vi "(SubVI)-Cut and Fit to Sutckbead-XY-QPD&BeadPosition_YCC.vi"(5 "Stuckbead path (dialog if empty)":path) -> (0 "Best Fit for Bead position (nm)":dbl[](array[numeric]), 1 "Cut-BeadPosition Array Out (nm)":dbl[](array[numeric]), 2 "Cut-QPD signal Out":dbl[](array[numeric]), 3 "All fig":T2(array[cluster]), 4 "Polynomial Coefficients\nx:QPD, y:BeadPos":dbl[](array[numeric]))   [LabVIEW 2014]
uses:
  <vilib>/Utility/file.llb/Read From Spreadsheet File (DBL).vi
  <vilib>/Analysis/NI_AALPro.lvlib
panel:
  out "XY Graph 2":T1(graph)
  out "XY Graph":T2(graph)
  out "stuckbead-QPD (V)":dbl[](array[numeric])
  out "Stage (um)":dbl[](array[numeric])
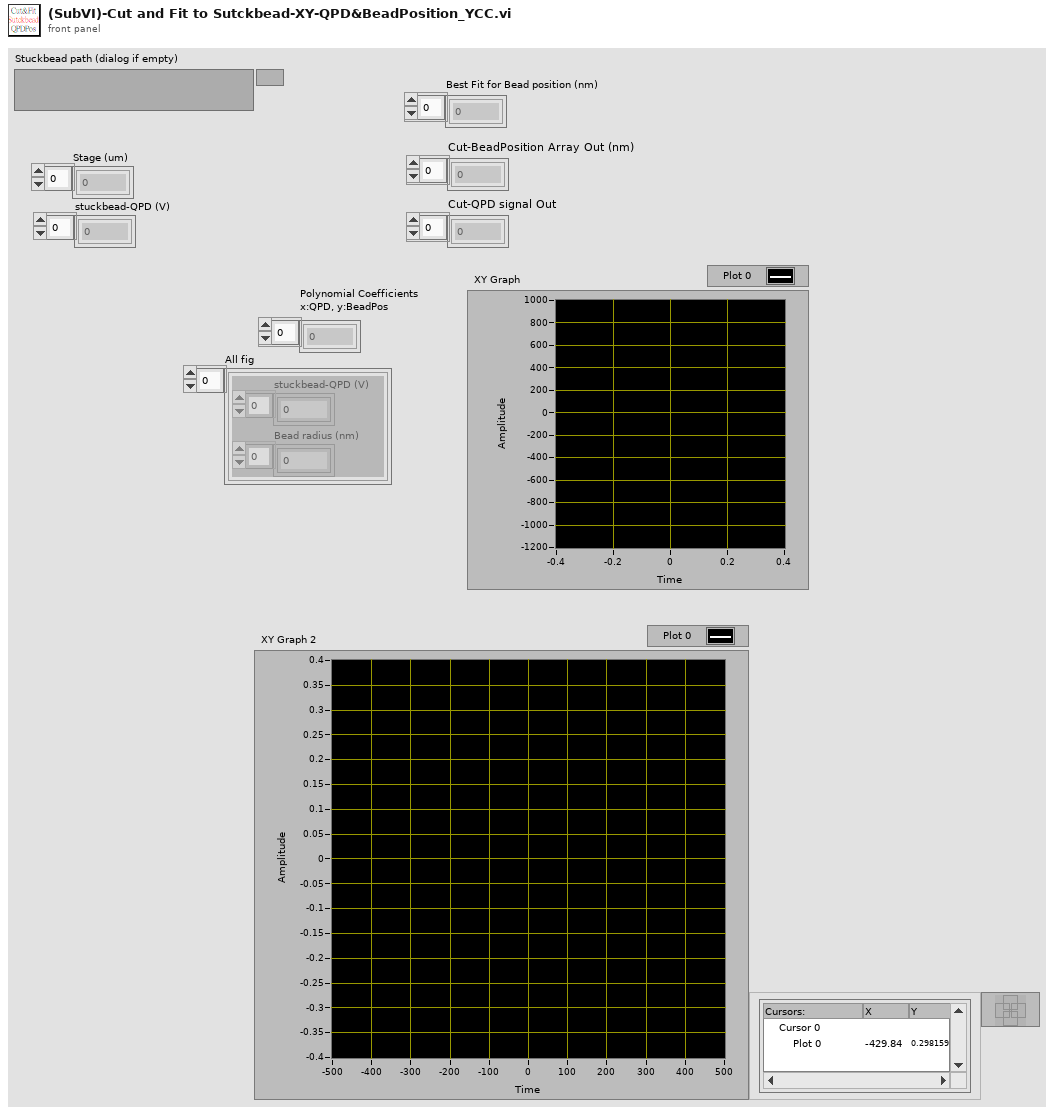
[diagram p1: front panel]
types:
  T1 = cluster{"Bead radius (nm)":dbl[], "Aligned QPD (V)":dbl[]}
  T2 = cluster{"stuckbead-QPD (V)":dbl[], "Bead radius (nm)":dbl[]}[]
  T3 = cluster{"QPD signal Out":dbl[], "Best Polynomial Fit":dbl[]}
  T4 = cluster{"QPD signal Out":dbl[], "Position Array Out":dbl[]}
  T5 = cluster{"stuckbead-QPD (V)":dbl[], "Bead radius (nm)":dbl[]}
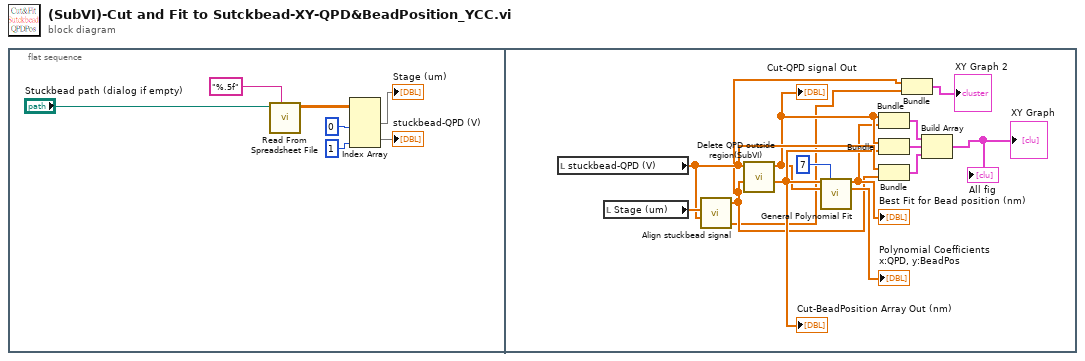
[diagram p0: block diagram]
diagram:
  n1 = flat-sequence {
    frame #0 {
      n2 = call-poly <vilib>:"Read From Spreadsheet File.vi"("format (%.3f)"="%.5f", "file path (dialog if empty)"="Stuckbead path (dialog if empty)") -> ("all rows"=w5:dbl[][])  [unwired: 5 in, 4 out]
      n3 = Index Array(array=w5, index (col) #1=0 ("disabled index (col)"), index (col) #2=1 ("disabled index (col)")) -> (element #1=→"Stage (um)":dbl[], element #2=→"stuckbead-QPD (V)":dbl[])  [unwired: 2 in]
    }
    frame #1 {
      n4 = local read "stuckbead-QPD (V)"() -> (w18:dbl[])
      n5 = local read "Stage (um)"() -> (w21:dbl[])
      n6 = call "Align stuckbead signal.vi"("stuckbstuck QPD (V)"=w18, "Stage (um)"=w21) -> ("Aligned QPD (V)"=w9:dbl[], "Bead radius (nm)"=w10:dbl[])  [unwired: 3 in]
      n7 = call "Delete QPD outside region(SubVI).vi"("Position Array In"=w10, "QPD signal In"=w18) -> ("Position Array Out"=w17:dbl[], "QPD signal Out"=w16:dbl[])  [unwired: 8 in]
      "Cut-QPD signal Out" <- w16
      "Cut-BeadPosition Array Out (nm)" <- w17
      n8 = call <vilib>:"General Polynomial Fit.vi"("Y"=w17, "polynomial order"=7, "X"=w16) -> ("Best Polynomial Fit"=w15:dbl[], "Polynomial Coefficients"=→"Polynomial Coefficients\nx:QPD, y:BeadPos":dbl[])  [unwired: 9 in, 2 out]
      "Best Fit for Bead position (nm)" <- w15
      n9 = Bundle("QPD signal Out"=w16, "Best Polynomial Fit"=w15) -> (w14:T3)  [unwired: 1 in]
      n10 = Bundle("QPD signal Out"=w16, "Position Array Out"=w17) -> (w13:T4)  [unwired: 1 in]
      n11 = Bundle("stuckbead-QPD (V)"=w18, "Bead radius (nm)"=w10) -> (w12:T5)  [unwired: 1 in]
      n12 = Bundle("Bead radius (nm)"=w10, "Aligned QPD (V)"=w9) -> (→"XY Graph 2":T1)  [unwired: 1 in]
      n13 = Build Array(w14, w13, w12) -> (→"XY Graph" →"All fig":T2)
    }
  }
